vi "verify waveplate_pos.vi"(8 "error in (no error)":errorcluster, 11 "SPARC4_Channel in":refnum<class "SPARC4_Channel.lvclass">) -> (0 "error out":errorcluster, 3 "SPARC4_Channel out":refnum<class "SPARC4_Channel.lvclass">)   [LabVIEW 2018, in "SPARC4_Channel.lvclass"]
uses:
  SPARC4_Channel.lvclass
  C:/Users/Denis/Desktop/S4ACS/S4ACS/Channel/Channel.lvclass
  Channel/Channel.lvclass/Channel.ctl
  SPARC4_Channel.lvclass/SPARC4_Channel.ctl
  Channel/Channel.lvclass
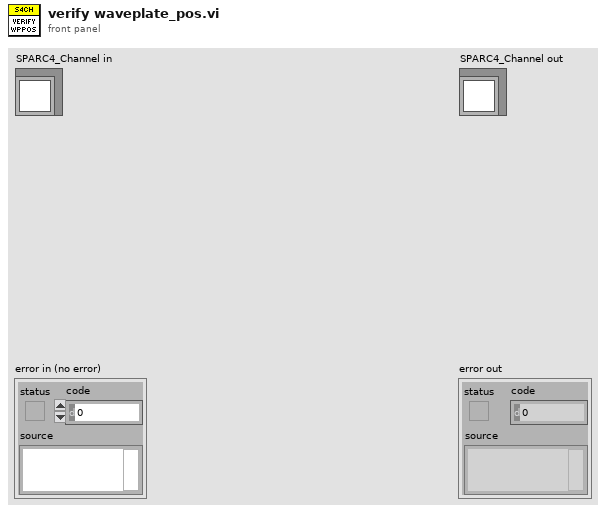
[diagram p1: front panel]
types:
  T1 = cluster{"#CYCLES":errorcluster, "SUFFIX":errorcluster}
  T2 = cluster{"#SEQS":errorcluster, "WAVEPLATE_POS":errorcluster}
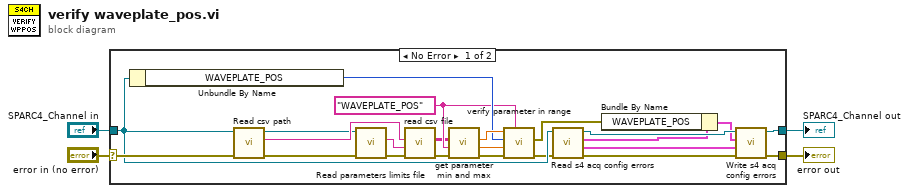
[diagram p0: block diagram]
diagram:
  n1 = case shown="No Error" "error in (no error)" {
    selector: "error in (no error)" -> [w20 w29]
    tunnel: [w11 w29] -> w3
    tunnel: [w12 w28] -> w1
    tunnel: "SPARC4_Channel in" -> [w14 w28]
    frame No Error {
      w24 = "WAVEPLATE_POS" ("parameter name")
      n2 = Unbundle By Name(w14) -> ("WAVEPLATE_POS"=w25:i32)
      n3 = call "Read csv path.vi"("error in (no error)"=w20, "Channel in"=w14) -> ("error out"=w19:errorcluster, "csv path"=w16:string, "Channel out"=w15:refnum<class "SPARC4_Channel.lvclass">)  [unwired: 7 in]
      n4 = call "Read parameters limits file.vi"("error in (no error)"=w19, "Channel in"=w15) -> ("error out"=w18:errorcluster, "parameters limits file"=w17:string)  [unwired: 7 in, 1 out]
      n5 = call "read csv file.vi"("error in"=w18, "file name"=w17, "file path"=w16) -> ("error out"=w22:errorcluster, "csv array"=w23:string[][])  [unwired: 7 in]
      n6 = call "get parameter min and max.vi"("error in (no error)"=w22, "parameter name"=w24, "limit values"=w23) -> ("error out"=w21:errorcluster, "min"=w27:dbl, "max"=w26:dbl)  [unwired: 6 in]
      n7 = call "verify parameter in range.vi"("parameter name"=w24, "error in (no error)"=w21, "lower limit"=w27, "value"=w25, "upper limit"=w26) -> ("error out"=w9:errorcluster, "verific error"=w5:errorcluster)  [unwired: 5 in]
      n8 = call "Read s4 acq config errors.vi"("error in (no error)"=w9, "SPARC4_Channel in"=w14) -> ("error out"=w10:errorcluster, "acquisition config errors"=w6:T1, "s4 acq config errors"=w8:T2, "SPARC4_Channel out"=w13:refnum<class "SPARC4_Channel.lvclass">)  [unwired: 6 in]
      n9 = Bundle By Name(cluster=w8, "WAVEPLATE_POS"=w5) -> (w7:T2)
      n10 = call "Write s4 acq config errors.vi"("error in (no error)"=w10, "acquisition config errors"=w6, "s4 acq config errors"=w7, "SPARC4_Channel in"=w13) -> ("error out"=w11:errorcluster, "SPARC4_Channel out"=w12:refnum<class "SPARC4_Channel.lvclass">)  [unwired: 6 in]
    }
    frame Error {
    }
  }
  "error out" <- w3
  "SPARC4_Channel out" <- w1
